vi "LVPortSetNamepathValue.vi"(8 "Error in":errorcluster, 9 "ObjectMap":T1[](array[typedef]), 10 "Object ID":i32, 11 "pID":string) -> (0 "Error out":errorcluster, 2 "Updated count":dbl, 3 "Object ID (Validated)":i32)   [LabVIEW 2017]
uses:
  Common/ObjectMap/LVPortObjectMapNamepathData.ctl
  Common/ObjectMap/LVPortObjectMapDataTypeEnum.ctl
  Common/ObjectMap/LVPortObjectMapContainerTypeEnum.ctl
  Common/ObjectMap/LVPortObjectMapDefaultIDsEnum.ctl
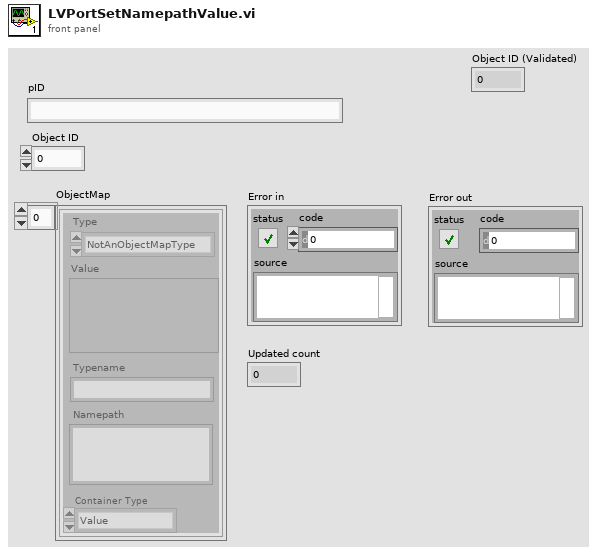
[diagram p1: front panel]
types:
  T1 = typedef "LVPortObjectMapNamepathData.ctl" = cluster{"Type":T2, "Value":variant, "Namepath":string, "Typename":string, "Container Type":T3}
  T2 = typedef "LVPortObjectMapDataTypeEnum.ctl" = enum16{"NotAnObjectMapType", "Real", "Complex", "String", "Boolean"}
  T3 = typedef "LVPortObjectMapContainerTypeEnum.ctl" = enum16{"Value", "Array", "Waveform"}
  T4 = typedef "LVPortObjectMapDefaultIDsEnum.ctl" = i32
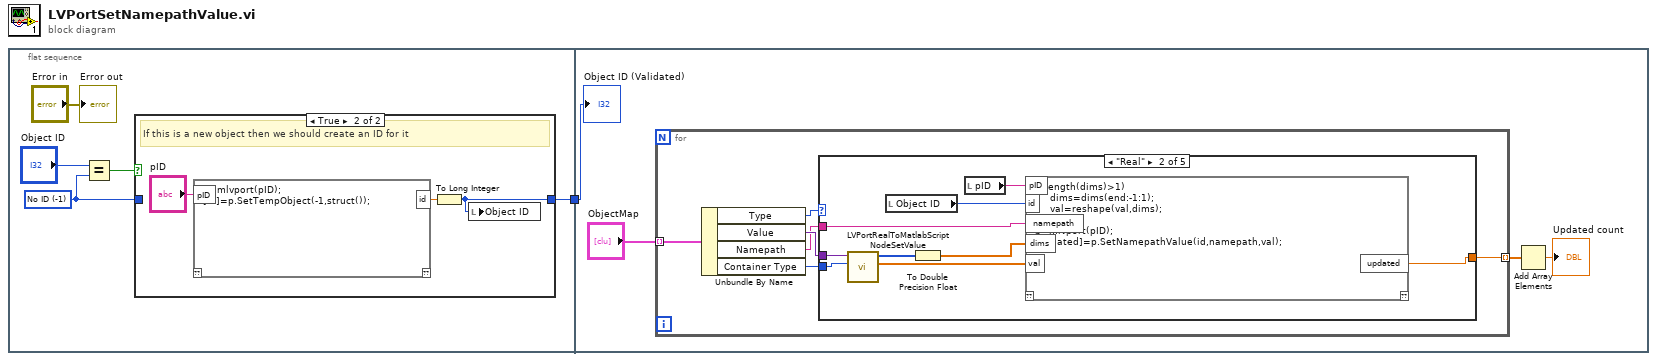
[diagram p0: block diagram]
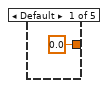
[diagram p3: hidden frame]
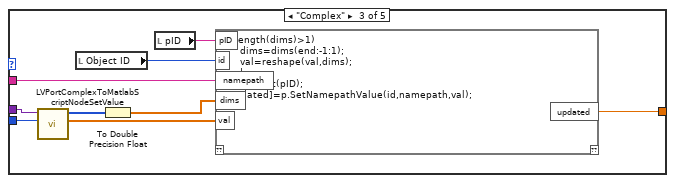
[diagram p4: hidden frame]
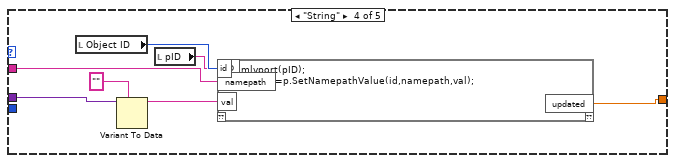
[diagram p5: hidden frame]
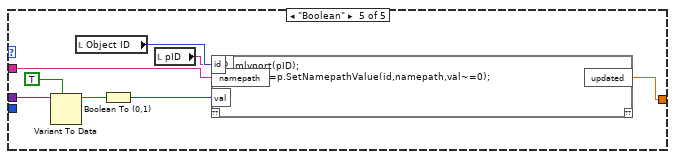
[diagram p6: hidden frame]
diagram:
  n1 = flat-sequence {
    tunnel: [w3] -> w1
    tunnel: w1 -> [w11]
    frame #0 {
      w4 = T4 -1 items=["No ID"=-1, "Port Object"=-2] ("Default IDs")
      n2 = Equal?(x="Object ID", y=w4) -> (x = y?=w6:bool)
      n3 = case shown="True" w6 {
        tunnel: w4 -> [w7 _]
        tunnel: [w7 w8] -> w3
        frame False {
        }
        frame True {
          # "If this is a new object then we should create an ID for it"
          n4 = script code="p=mlvport(pID);\n[id]=p.SetTempObject(-1,struct());"("pID"="pID") -> ("id"=w9:dbl)  [unwired: 1 in, 1 out]
          n5 = To Long Integer(number=w9) -> (32bit integer=w8:i32)
          n6 = local write "Object ID"(w8) -> ()
        }
      }
      "Error out" <- "Error in"
    }
    frame #1 {
      n7 = for {
        tunnel: "ObjectMap" -> [w20] mode=indexing
        tunnel: [w15] -> w13 mode=indexing
        n8 = Unbundle By Name(w20) -> ("Type"=w18:T2, "Value"=w17:variant, "Namepath"=w16:string, "Container Type"=w19:T3)
        n9 = case shown="\"Real\"" w18 {
          tunnel: w16 -> [_ w30 w39 w46 w51]
          tunnel: w19 -> [_ w26 w35 _ _]
          tunnel: w17 -> [_ w25 w34 w44 w50]
          tunnel: [0.0 w22 w31 w40 w47] -> w15
          frame Default {
          }
          frame "Real" {
            n10 = call "LVPortRealToMatlabScriptNodeSetValue.vi"("Container Type"=w26, "Value"=w25) -> ("1D Array"=w29:dbl[], "Size(s)"=w28:u32[])  [unwired: 8 in]
            n11 = local read "Object ID"() -> (w23:i32)
            n12 = To Double Precision Float(number=w28) -> (double precision float=w27:dbl[])
            n13 = local read "pID"() -> (w24:string)
            n14 = script code="if(length(dims)>1)\n     dims=dims(end:-1:1);\n     val=reshape(val,dims);\nend\np=mlvport(pID);\n[updated]=p.SetNamepathValue(id,namepath,val);"("pID"=w24, "namepath"=w30, "val"=w29, "dims"=w27, "id"=w23) -> ("updated"=w22:dbl)  [unwired: 1 in, 1 out]
          }
          frame "Complex" {
            n15 = call "LVPortComplexToMatlabScriptNodeSetValue.vi"("Container Type"=w35, "Value"=w34) -> ("1D Array"=w38:cdb[], "Size(s)"=w37:u32[])  [unwired: 8 in]
            n16 = local read "Object ID"() -> (w32:i32)
            n17 = To Double Precision Float(number=w37) -> (double precision float=w36:dbl[])
            n18 = local read "pID"() -> (w33:string)
            n19 = script code="if(length(dims)>1)\n     dims=dims(end:-1:1);\n     val=reshape(val,dims);\nend\np=mlvport(pID);\n[updated]=p.SetNamepathValue(id,namepath,val);"("pID"=w33, "namepath"=w39, "val"=w38, "dims"=w36, "id"=w32) -> ("updated"=w31:dbl)  [unwired: 1 in, 1 out]
          }
          frame "String" {
            n20 = local read "Object ID"() -> (w42:i32)
            n21 = Variant To Data(type="" ("Name"), Variant=w44) -> (data=w45:string)  [unwired: 1 in, 1 out]
            n22 = local read "pID"() -> (w41:string)
            n23 = script code="p=mlvport(pID);\n[updated]=p.SetNamepathValue(id,namepath,val);"("pID"=w41, "namepath"=w46, "val"=w45, "id"=w42) -> ("updated"=w40:dbl)  [unwired: 1 in, 1 out]
          }
          frame "Boolean" {
            n24 = Variant To Data(type=TRUE, Variant=w50) -> (data=w53:bool)  [unwired: 1 in, 1 out]
            n25 = local read "Object ID"() -> (w49:i32)
            n26 = Boolean To (0,1)(Boolean=w53) -> (0, 1=w52:i16)
            n27 = local read "pID"() -> (w48:string)
            n28 = script code="p=mlvport(pID);\n[updated]=p.SetNamepathValue(id,namepath,val~=0);"("pID"=w48, "namepath"=w51, "val"=w52, "id"=w49) -> ("updated"=w47:dbl)  [unwired: 1 in, 1 out]
          }
        }
      }
      n29 = Add Array Elements(numeric array=w13) -> (sum=→"Updated count":dbl)
      "Object ID (Validated)" <- w11
    }
  }
